vi "setValue.vi"(8 "error in (no error)":errorcluster, 10 "String":string, 11 "tBSONString in":refnum<class "tBSONString.lvclass">) -> (0 "error out":errorcluster, 3 "tBSONString out":refnum<class "tBSONString.lvclass">)   [LabVIEW 2013, in "BSON.lvlib" / "tBSONString.lvclass"]
uses:
  tBSONString.lvclass
  tBSONString.lvclass/tBSONString.ctl
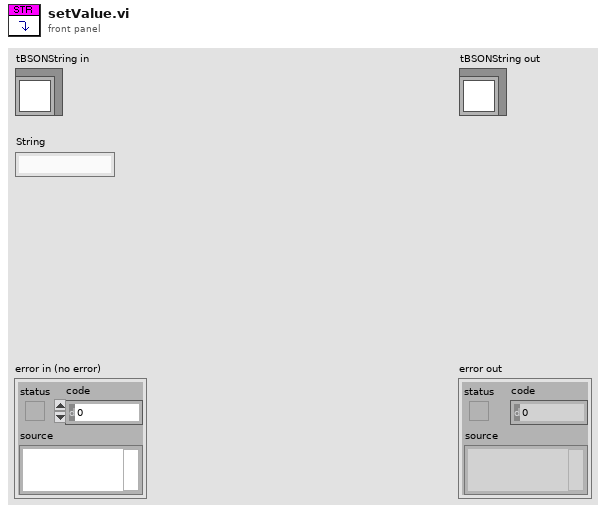
[diagram p1: front panel]
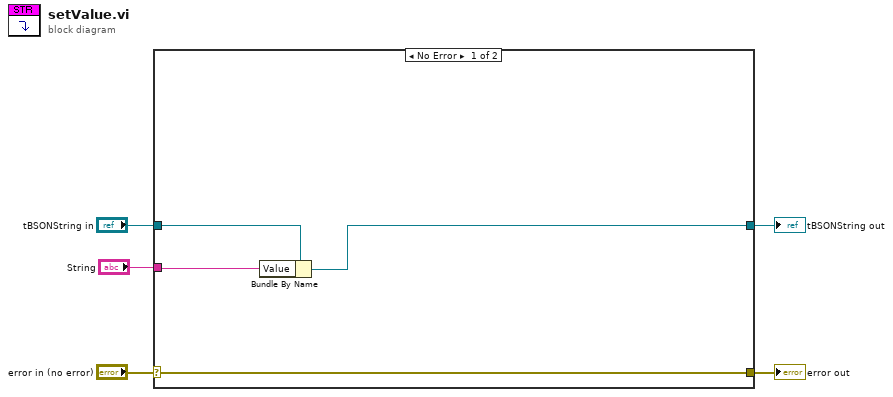
[diagram p0: block diagram]
diagram:
  n1 = case shown="No Error" "error in (no error)" {
    selector: "error in (no error)" -> [w9 w11]
    tunnel: [w9 w11] -> w4
    tunnel: [w6 w10] -> w2
    tunnel: "tBSONString in" -> [w8 w10]
    tunnel: "String" -> [w7 _]
    frame No Error {
      n2 = Bundle By Name(cluster=w8, "Value"=w7) -> (w6:refnum<class "tBSONString.lvclass">)
    }
    frame Error {
    }
  }
  "error out" <- w4
  "tBSONString out" <- w2
